vi "Process.vi"(8 "error in":errorcluster, 11 "Inst UI.MOTOR":refnum<class "Inst UI.MOTOR.lvclass">) -> (0 "error out":errorcluster, 3 "Inst UI.MOTOR out":refnum<class "Inst UI.MOTOR.lvclass">)   [LabVIEW 2019, in "Inst UI.MOTOR.lvclass"]
doc: "---------------------------------------------------------------\nJKI State Machine Objects™\nhttp://jki.net/state-machine-objects/\nCopyright (C) 2005-2015, JKI <info@jki.net>\nALL RIGHTS RESERVEDJKI State Machine Objects (SMO) 1.0.0.5\nJKI - JKI\nCopyright (c) 2016, JKI"
uses:
  Inst UI.MOTOR.lvclass
  C:/Program Files (x86)/National Instruments/LabVIEW 2019/vi.lib/JKI/JKI SMO/SMO/SMO.lvclass
  C:/Program Files (x86)/National Instruments/LabVIEW 2019/user.lib/LevyLab/Instrument Framework/SMOs/Instrument UI/Instrument UI.lvclass
  C:/Program Files (x86)/National Instruments/LabVIEW 2019/vi.lib/JKI/JKI SMO/SMO.UI/SMO.UI.lvclass
  Motor/Serial - XON-XOFF Characters.ctl
  Motor/Serial - ASCII Characters.ctl
  Inst.MOTOR/Typedefs/Inst.MOTOR.Commands--Enum.ctl
  Inst.MOTOR/Typedefs/Inst.MOTOR.getAll--Cluster.ctl
  Inst.MOTOR/Inst.MOTOR.lvclass
  C:/Program Files (x86)/National Instruments/LabVIEW 2019/user.lib/LevyLab/Instrument Framework/SMOs/Instrument/Instrument.lvclass
  Inst UI.MOTOR.UI--Cluster.ctl
  <userlib>/LevyLab/Instrument Framework/SMOs/Configuration/Configuration.lvclass
  <userlib>/LevyLab/Instrument Framework/SMOs/RemoteControl/Typedefs/Message--Cluster.ctl
  Inst.MOTOR/Typedefs/Inst.MOTOR.Configuration--Cluster.ctl
  <userlib>/LevyLab/Instrument Framework/SMOs/Instrument UI/Instrument UI.lvclass/Instrument UI.ctl
  Inst.MOTOR/Inst.MOTOR.lvclass/Inst.MOTOR.ctl
  <vilib>/JKI/JKI SMO/SMO/SMO.lvclass/SMO.ctl
  <userlib>/LevyLab/Instrument Framework/SMOs/Configuration/Configuration.lvclass/Configuration.ctl
  <userlib>/LevyLab/Instrument Framework/SMOs/Instrument/Instrument.lvclass/Instrument.ctl
  <userlib>/LevyLab/Instrument Framework/SMOs/Instrument/Typedefs/Client Type--Enum.ctl
  09e9697b-516c-49fb-b2dc-692589121b6f.vi
  <vilib>/JKI/JKI SMO/SMO/Private/ReftoDVR--SMO.vi
  09e9697b-516c-49fb-b2dc-692589121b6f.vi/bd16e97c-1283-4bf0-81fa-9ddf6985c1ae.vi
  09e9697b-516c-49fb-b2dc-692589121b6f.vi/bd16e97c-1283-4bf0-81fa-9ddf6985c1ae.vi/4ce74e04-6dcf-45ed-9e3a-8688fabe3fd2.vi
  <userlib>/LevyLab/Instrument Framework/SMOs/Instrument/API/Send and Receive.vi
  09e9697b-516c-49fb-b2dc-692589121b6f.vi/bd16e97c-1283-4bf0-81fa-9ddf6985c1ae.vi/122f345b-9992-4887-9e4c-64365b80683c.vi
  <userlib>/LevyLab/Instrument Framework/SMOs/Instrument/Private/Get Client Type.vi
  09e9697b-516c-49fb-b2dc-692589121b6f.vi/bd16e97c-1283-4bf0-81fa-9ddf6985c1ae.vi/4ce74e04-6dcf-45ed-9e3a-8688fabe3fd2.vi/d12c5baa-aee5-401d-8272-1247450cc591.vi
  09e9697b-516c-49fb-b2dc-692589121b6f.vi/bd16e97c-1283-4bf0-81fa-9ddf6985c1ae.vi/4ce74e04-6dcf-45ed-9e3a-8688fabe3fd2.vi/9d50bdb1-c95d-42e6-b665-6d4980af7bdd.vi
  09e9697b-516c-49fb-b2dc-692589121b6f.vi/bd16e97c-1283-4bf0-81fa-9ddf6985c1ae.vi/122f345b-9992-4887-9e4c-64365b80683c.vi/c58dab05-969e-483a-9f90-fe9d022133c9.vi
  09e9697b-516c-49fb-b2dc-692589121b6f.vi/bd16e97c-1283-4bf0-81fa-9ddf6985c1ae.vi/122f345b-9992-4887-9e4c-64365b80683c.vi/09663c29-364a-4026-bee6-568e439f1e9d.vi
  09e9697b-516c-49fb-b2dc-692589121b6f.vi/bd16e97c-1283-4bf0-81fa-9ddf6985c1ae.vi/122f345b-9992-4887-9e4c-64365b80683c.vi/c58dab05-969e-483a-9f90-fe9d022133c9.vi/7baa1985-5e51-47ea-8afb-6dd3369df49d.vi
  09e9697b-516c-49fb-b2dc-692589121b6f.vi/bd16e97c-1283-4bf0-81fa-9ddf6985c1ae.vi/122f345b-9992-4887-9e4c-64365b80683c.vi/c58dab05-969e-483a-9f90-fe9d022133c9.vi/1d83d098-8c96-44ae-b21b-eeb7af13dafe.vi
  <userlib>/LevyLab/Instrument Framework/SMOs/Instrument/Private/Get RC Connection Status.vi
  <userlib>/LevyLab/Instrument Framework/SMOs/RemoteControl/API/Send and Receive.vi
  <vilib>/Utility/Data Type/Get Type Information.vi
  <vilib>/JDP Science/JSONtext/JSON text to Variant.vi
  <vilib>/JDP Science/JSONtext/Variant to JSON Text.vi
  <vilib>/National Instruments/GUID Generator/Guid Generator.vi
  <userlib>/LevyLab/Instrument Framework/SMOs/Instrument/Private/Instrument.MessageFromProcess.EventStructure.vi
  <userlib>/LevyLab/Instrument Framework/SMOs/Instrument/Instrument.lvclass
  <vilib>/JDP Science/JSONtext/LVClass Serializer/JSONtext LVClass Serializer.lvclass
  <userlib>/LevyLab/Instrument Framework/SMOs/Instrument UI/Instrument UI.lvclass
  <vilib>/JKI/JKI SMO/SMO/SMO.lvclass
  <vilib>/JKI/JKI SMO/SMO.UI/SMO.UI.lvclass
  <userlib>/LevyLab/Instrument Framework/SMOs/RemoteControl/RemoteControl.lvclass
  C:/Program Files (x86)/National Instruments/LabVIEW 2019/user.lib/LevyLab/Instrument Framework/Instrument Types/VSource/Instrument.VSource.lvclass
panel:
  out "Encoder Position":string
  in  "Tab Control":T1(tab)
  in  "Encoder Position":bool
  in  "Choose wfm":string(combo)
  in  "Stop Motor":bool
  in  "Set Encoder Data":bool
  in  "Set Jog":bool
  in  "wfmStep":i32
  in  "uStep":i32
  in  "Speed":i32
  in  "Angle":i32
  in  "Target Mode":bool
  in  "Speed":i32
  in  "Write Command":string="*IDN?"
  in  "Write":bool
  in  "Read":bool
  out "coerced(x)":u32
  out "Response":string
  in  "XON/XOFF Characters":T2={"XON"=enum."DC1", "XOFF"=enum."DC3"}
  in  "STOP":bool
  # "MOTOR"
  # "For instructions on how to use the JKI State Machine Objects, examples and video tutorials, visit:\nhttp://jki.net/state-machine-objects/\n\nJKI State Machine Objects™\nhttp://jki.net/state-machine-objects/\nCopyright (C) 2005-2015, JKI <info@jki.net>\nALL RIGHTS RESERVED"
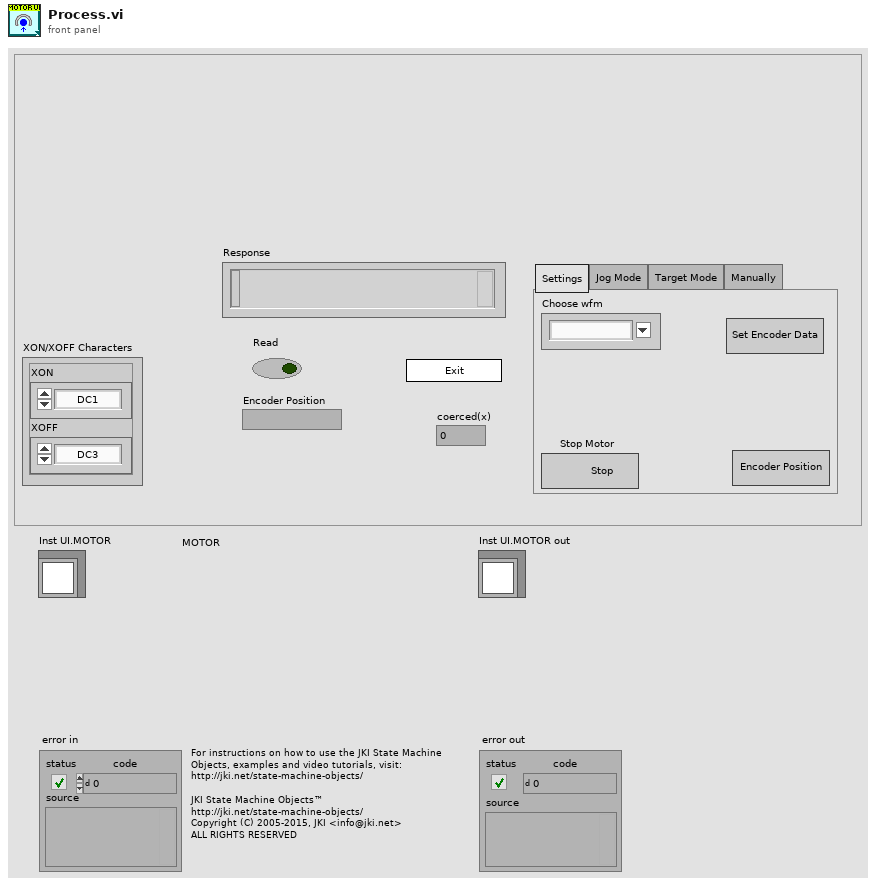
[diagram p1: front panel]
types:
  T1 = enum32{"Settings", "Jog Mode", "Target Mode", "Manually"}
  T2 = typedef "Serial - XON-XOFF Characters.ctl" = cluster{"XON":T3, "XOFF":T3}
  T3 = typedef "Serial - ASCII Characters.ctl" = enum16{"NUL", "SOH", "STX", "ETX", "EOT", "ENQ", "ACK", "BEL", "BS", "HT", "LF", "VT", "FF", "CR", "SO", "SI", "DLE", "DC1", "DC2", "DC3", "DC4", "NAK", "SYN", "ETB", "CAN", "EM", "SUB", "ESC", "FS", "GS", "RS", "US", "SP", "!", "\"", "#", "$", "%", "&", "'", "(", ")", "*", "+", ",", "- (-)", ".", "/", "0", "1", "2", "3", "4", "5", "6", "7", "8", "9", ":", ";", "<", "=", ">", "?", "@", "A", "B", "C", "D", "E", "F", "G", "H", "I", "J", "K", "L", "M", "N", "O", "P", "Q", "R", "S", "T", "U", "V", "W", "X", "Y", "Z", "[", "\\", "]", "^", "_", "`", "a", "b", "c", "d", "e", "f", "g", "h", "i", "j", "k", "l", "m", "n", "o", "p", "q", "r", "s", "t", "u", "v", "w", "x", "y", "z", "{", "|", "}", "~"}
  T4 = typedef "Inst.MOTOR.lvclass/Inst.MOTOR.Commands--Enum.ctl" = enum16{"Encoder Position", "VISA Read", "VISA Write"}
  T5 = enum32{"invalid app kind", "Development System", "Run Time System", "Student Edition", "Embedded LabVIEW", "Evaluation", "Custom"}
  T6 = enum32{"Invalid", "Standard", "Closed", "Hidden", "Minimized", "Maximized"}
  T7 = typedef "Instrument.lvclass/Client Type--Enum.ctl" = enum16{"Remote", "Local"}
  T8 = typedef "RemoteControl.lvclass/Message--Cluster.ctl" = cluster{"Command":string, "Data":variant, "ID":string}
  T9 = typedef "Inst.MOTOR.lvclass/Inst.MOTOR.Configuration--Cluster.ctl" = cluster{"baud rate":u32, "data bits":u16, "parity":enum16{"None", "Odd", "Even", "Mark", "Space"}, "stop bits":u16, "flow control":u16, "Read Count":u32, "Address":refnum<visa-resource-name>, "Termination Character":u8}
  T10 = typedef "Inst.MOTOR.lvclass/Inst.MOTOR.getAll--Cluster.ctl" = cluster{"Response":string, "Forward":bool, "Stop Motor":bool, "Encoder Position":string}
  T11 = typedef "Inst UI.MOTOR.lvclass/Inst UI.MOTOR.UI--Cluster.ctl" = cluster{" Read":string, "VISA resource name":refnum<visa-resource-name>}
  T12 = cluster{"Core":cluster{"Current VI Reference":refnum<vi>, "Close Panel on Exit?":bool, "Last Error":cluster{"error":errorcluster, "previous state":string, "remaining states":string}, "Shutdown?":bool}, "Instrument UI":refnum<class "Inst UI.MOTOR.lvclass">, "Instrument":refnum<class "Inst.MOTOR.lvclass">, "Configuration":refnum<class "Configuration.lvclass">, "Config Cluster":T9, "getAll":T10, "UI Cluster":T11, "Message":T8}
  T13 = cluster{"Current VI Reference":refnum<vi>, "Close Panel on Exit?":bool, "Last Error":cluster{"error":errorcluster, "previous state":string, "remaining states":string}, "Shutdown?":bool}
  T14 = typedef "SMO.lvclass/Protected Events.ctl" = cluster{"StopProcesses":refnum<user-event>, "AbortProcesses":refnum<user-event>, "Config Changed":refnum<user-event>, "Dependency":refnum<user-event>}
  T15 = typedef "Instrument.lvclass/PublicEvents--Cluster.ctl" = cluster{"MessageFromProcess":refnum<user-event>}
  T16 = typedef "Inst.MOTOR.lvclass/PublicEvents--Cluster.ctl" = cluster{"MessageFromProcess":refnum<user-event>}
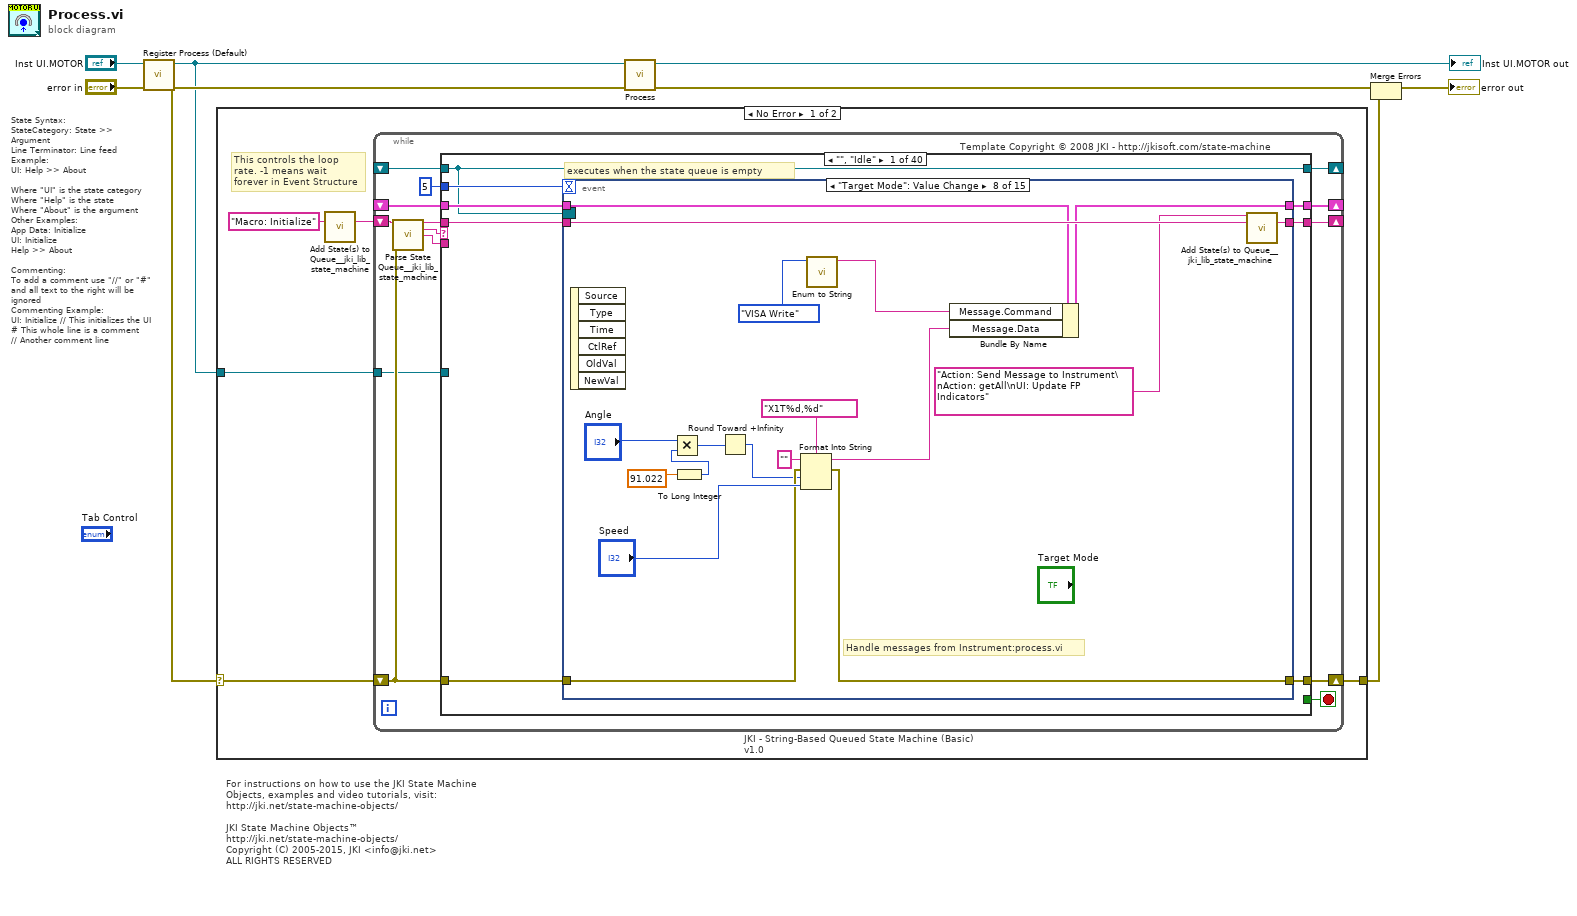
[diagram p0: block diagram]
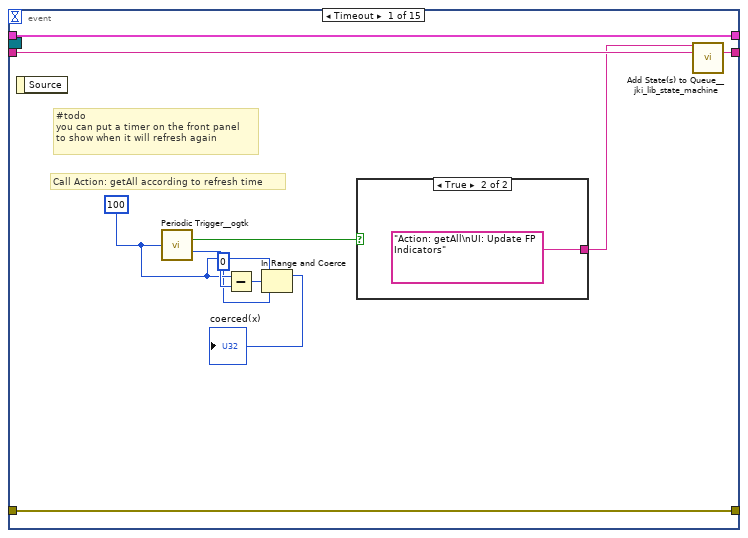
[diagram p2: hidden frame]
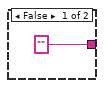
[diagram p3: hidden frame]
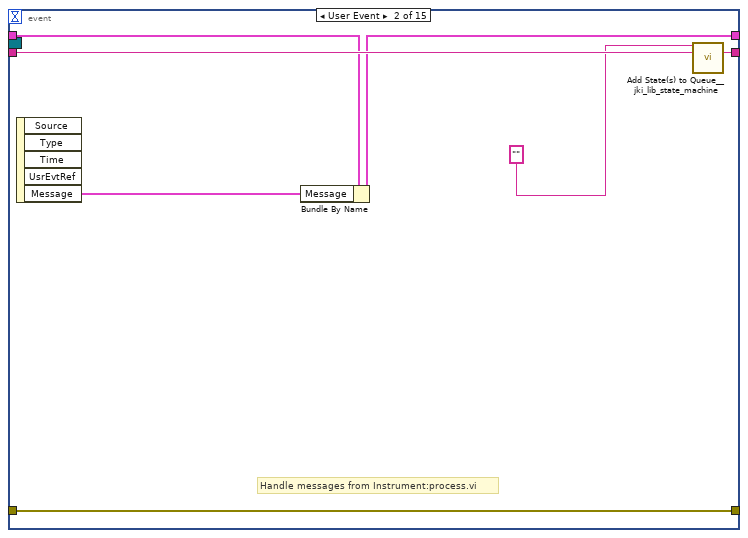
[diagram p4: hidden frame]
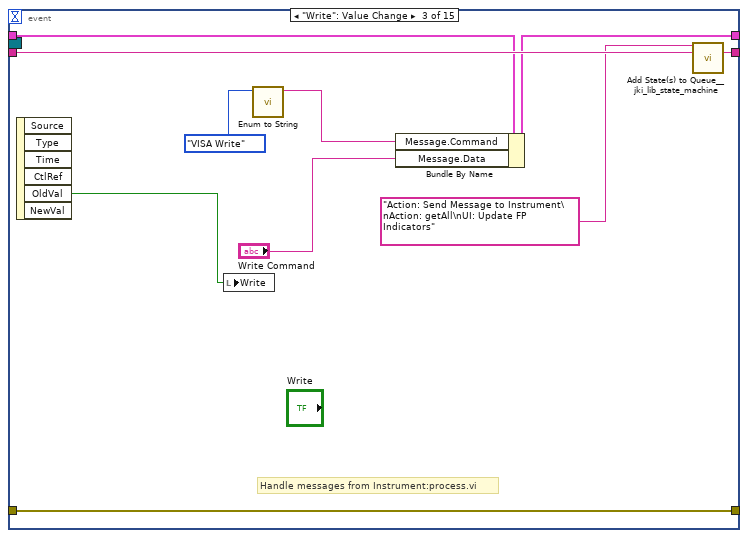
[diagram p5: hidden frame]
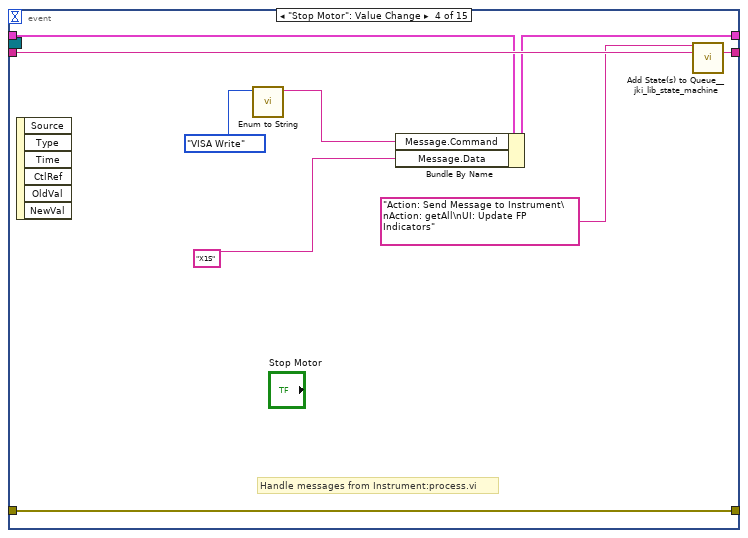
[diagram p6: hidden frame]
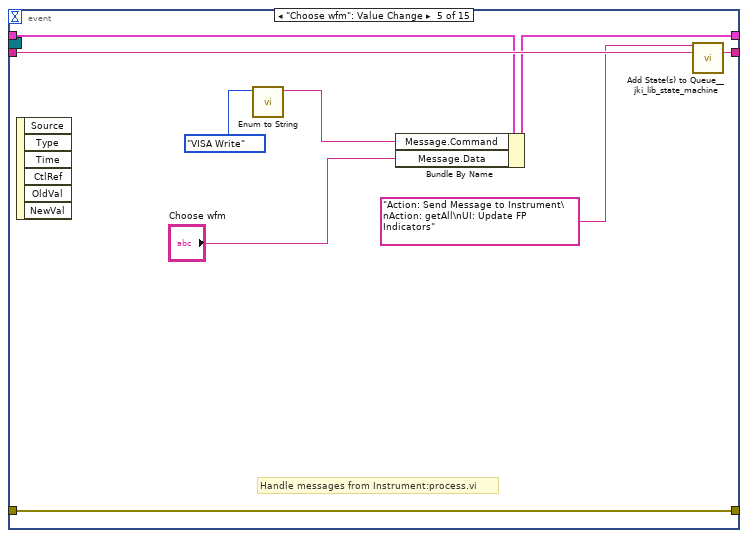
[diagram p7: hidden frame]
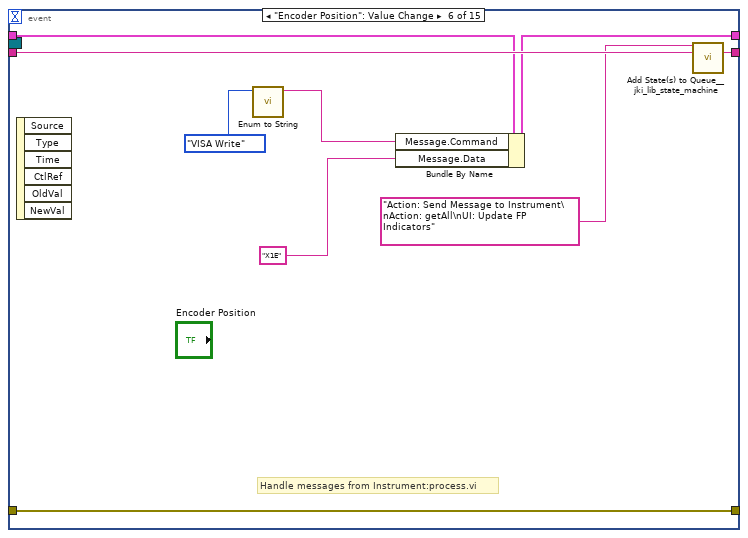
[diagram p8: hidden frame]
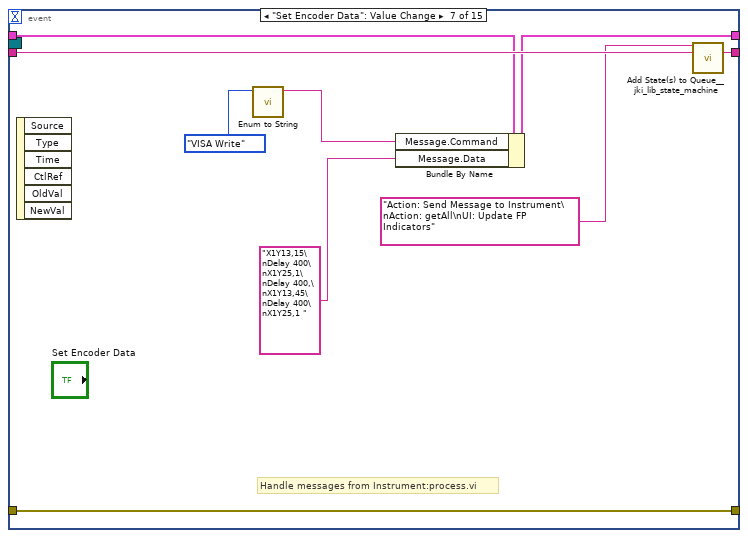
[diagram p9: hidden frame]
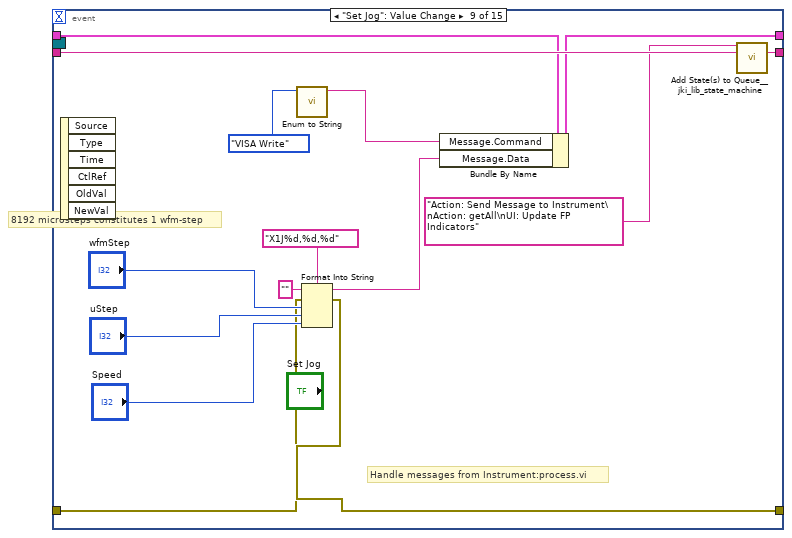
[diagram p10: hidden frame]
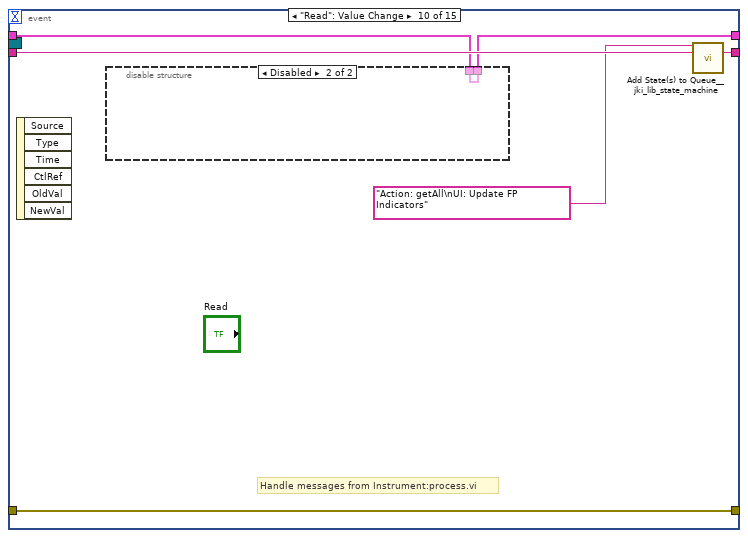
[diagram p11: hidden frame]
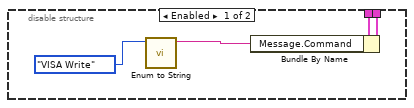
[diagram p12: hidden frame]
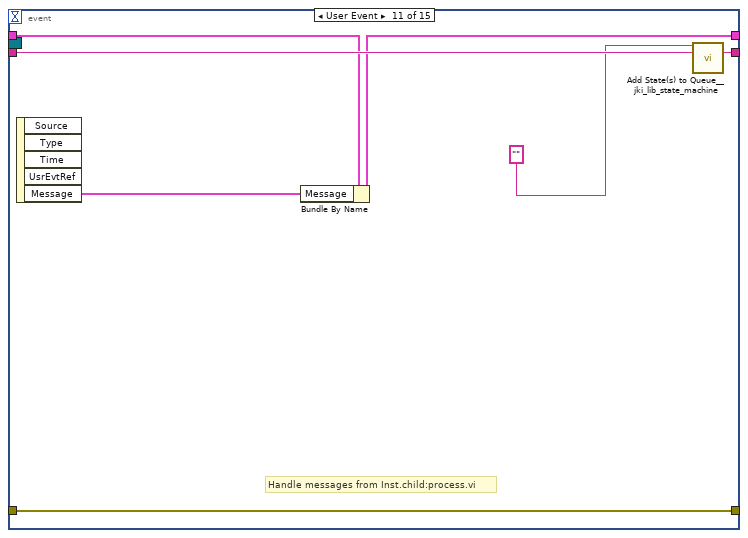
[diagram p13: hidden frame]
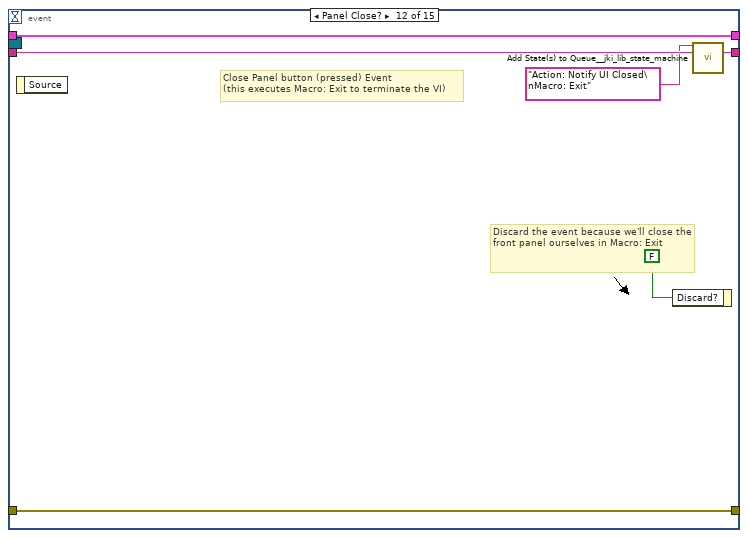
[diagram p14: hidden frame]
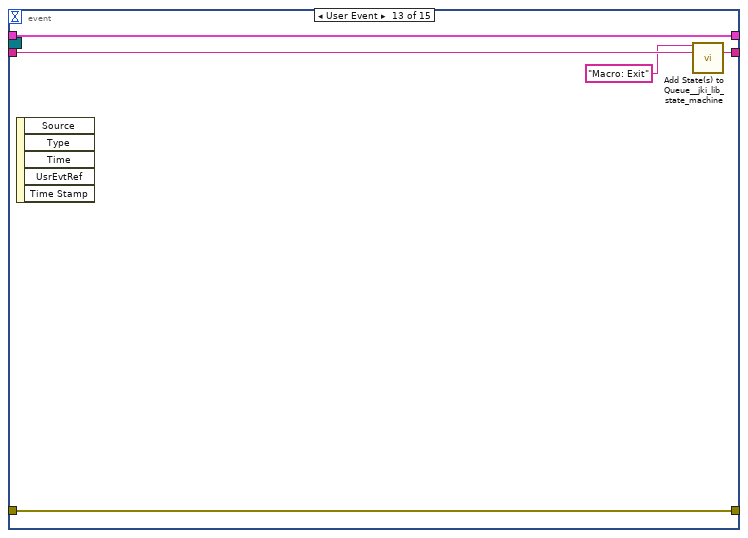
[diagram p15: hidden frame]
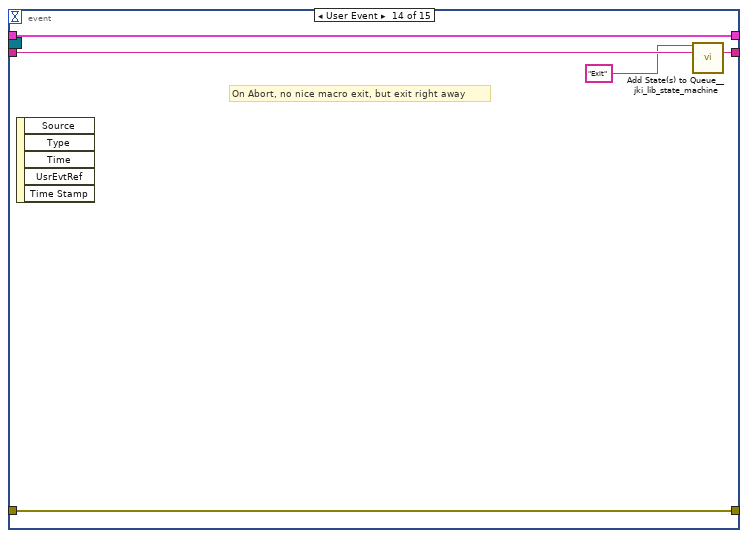
[diagram p16: hidden frame]
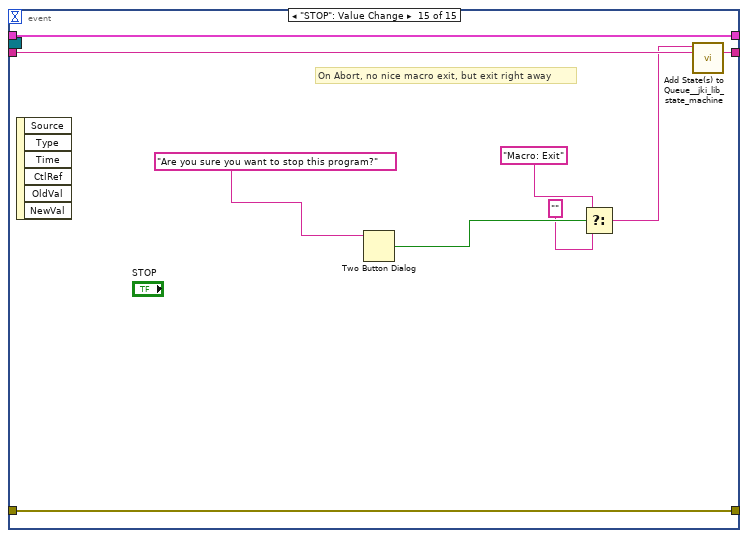
[diagram p17: hidden frame]
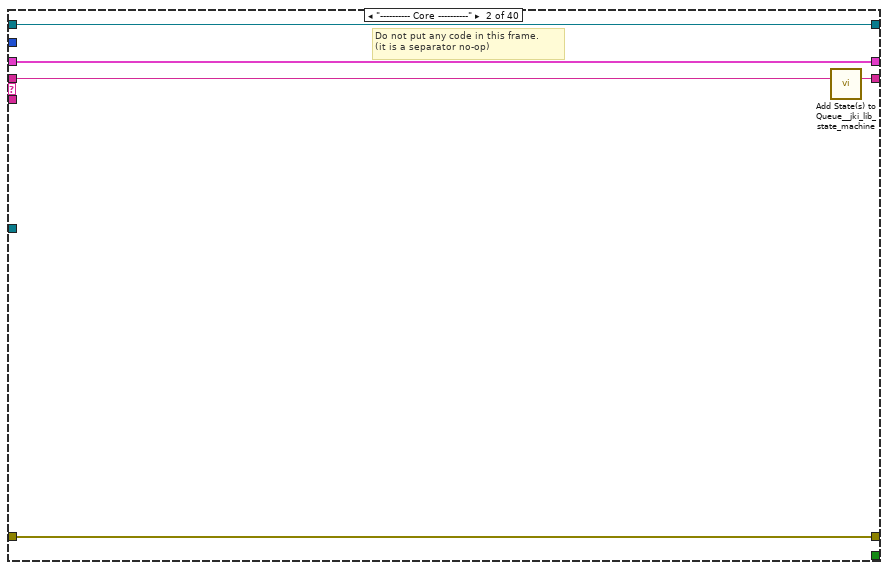
[diagram p18: hidden frame]
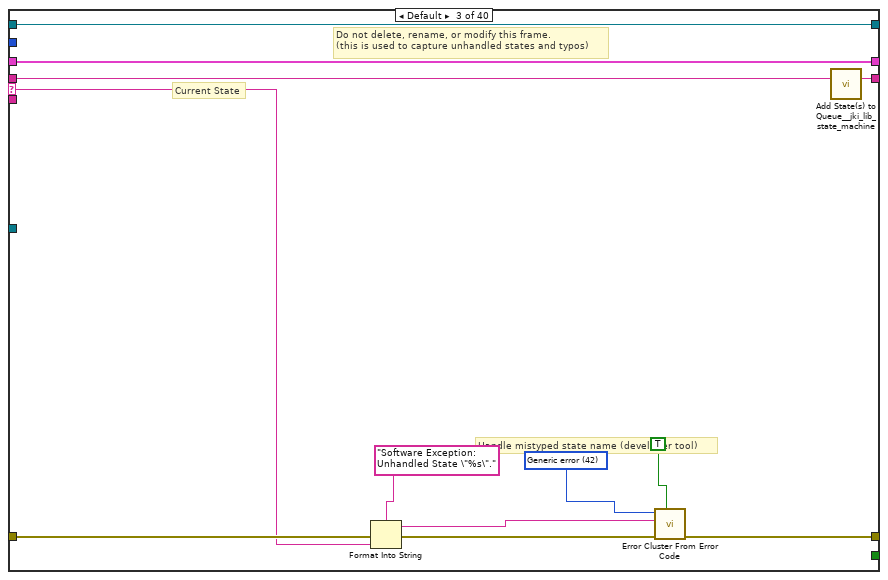
[diagram p19: hidden frame]
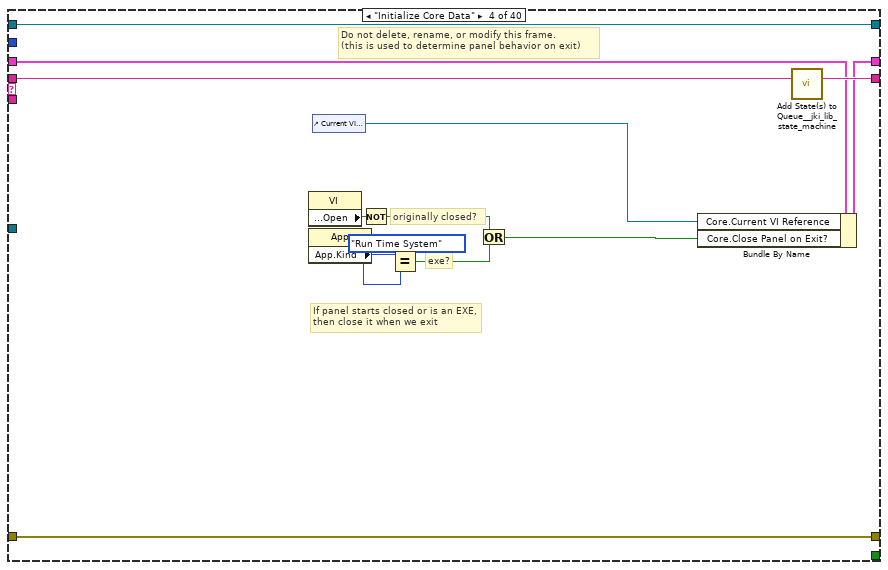
[diagram p20: hidden frame]
diagram:
  # "State Syntax:\nStateCategory: State >> Argument\nLine Terminator: Line feed\nExample:\nUI: Help >> About\n\nWhere \"UI\" is the state category\nWhere \"Help\" is the state\nWhere \"About\" is the argument\nOther Examples:\nApp Data: Initialize\nUI: Initialize\nHelp >> About\n\nCommenting:\nTo add a comment use \"//\" or \"#\" and all text to the right will be ignored\nCommenting Example:\nUI: Initialize // This initializes the UI\n# This whole line is a comment\n// Another comment line"
  # "For instructions on how to use the JKI State Machine Objects, examples and video tutorials, visit:\nhttp://jki.net/state-machine-objects/\n\nJKI State Machine Objects™\nhttp://jki.net/state-machine-objects/\nCopyright (C) 2005-2015, JKI <info@jki.net>\nALL RIGHTS RESERVED"
  n1 = call <vilib>:"Register Process (Default).vi"("error in (no error)"="error in", "SMO"="Inst UI.MOTOR") -> ("error out"=w5:errorcluster, "SelfRef"=w4:refnum<class "Inst UI.MOTOR.lvclass">)  [unwired: 8 in]
  n2 = case shown="No Error" w5 {
    selector: w5 -> [w10 w564]
    tunnel: w4 -> [w11 _]
    tunnel: [w9 w564] -> w1
    frame No Error {
      # "This controls the loop rate. -1 means wait forever in Event Structure"
      n3 = call <vilib>:"Add State(s) to Queue__jki_lib_state_machine.vi"("State(s) in (\"\")"="Macro: Initialize") -> ("States Out"=w13:string)  [unwired: 14 in]
      n4 = while "JKI - String-Based Queued State Machine (Basic) v1.0" {
        shift-right: [w20] -> _
        shift-left: _ -> [w19]
        shift-right: [w23] -> w9
        shift-left: w10 -> [w17]
        shift-right: [w22] -> _
        shift-left: w13 -> [w24]
        tunnel: w11 -> [w16]
        shift-right: [w15] -> _
        shift-left: _ -> [w14]
        stop <- w21 stop-if-true
        # "Template Copyright © 2008 JKI - http://jkisoft.com/state-machine"
        n5 = call <vilib>:"Parse State Queue__jki_lib_state_machine.vi"("State Queue"=w24, "Error In (no error)"=w17) -> ("Remaining States"=w26:string, "Current State"=w27:string, "Arguments"=w25:string)  [unwired: 11 in]
        n6 = case shown="\"\", \"Idle\"" w27 {
          selector: w27 -> [_ _ w184 _ _ _ _ _ _ _ _ _ _ _ _ _ _ _ _ _ _ _ _ _ _ _ _ _ _ _ _ _ _ _ _ _ _ _ _ _]
          tunnel: w26 -> [w35 w182 w188 w207 w211 w226 w231 w249 w254 w262 w269 w274 w281 w286 w295 w302 w318 w350 w359 w371 w381 w387 w402 w407 w418 w425 w430 w446 w452 w457 w472 w480 w492 w499 w506 w518 w531 w541 w553 w563]
          tunnel: w25 -> [_ _ _ _ _ _ _ _ _ _ _ _ _ _ _ w296 w312 _ _ _ _ _ _ _ _ _ _ _ _ _ _ _ _ _ _ _ _ _ _ _]
          tunnel: w19 -> [w33 w179 w186 w198 w214 w222 w228 _ w250 w258 w263 w271 w279 w283 w291 w300 w314 w347 w355 w361 w378 w384 w389 w404 w415 w420 w427 w444 w450 w454 w465 w477 w483 w494 w500 w510 w525 w533 w548 w558]
          tunnel: [w32 w180 w190 w204 w216 w221 w229 w238 w252 w260 w265 w272 w276 w282 w292 w297 w315 w348 w357 w369 w379 w385 w400 w405 w409 w421 w428 w441 w447 w455 w458 w475 w484 w496 w501 w515 w528 w538 w544 w554] -> w23
          tunnel: w17 -> [w31 w180 w189 w204 w210 _ w229 w235 w252 w260 w266 w272 w277 w282 w292 w298 w316 w348 w357 w369 w379 w385 w400 w405 w410 w422 w428 w431 w448 w455 w467 w473 w485 w496 w502 w511 w520 w534 w545 w555]
          tunnel: [w34 w181 w187 w206 w208 w225 w230 w248 w253 w261 w268 w273 w280 w285 w294 w301 w317 w349 w358 w370 w380 w386 w401 w406 w417 w424 w429 w445 w451 w456 w471 w479 w491 w498 w505 w517 w530 w540 w552 w562] -> w22
          tunnel: [_ _ _ _ _ TRUE _ _ _ _ _ _ _ _ _ _ _ _ _ _ _ _ _ _ _ _ _ _ _ _ _ _ _ _ _ _ _ _ _ _] -> w21
          tunnel: [w30 w179 w186 w205 w213 w222 w228 w247 w250 w258 w263 w271 w279 w283 w291 w300 w314 w347 w355 w362 w378 w384 w389 w404 w415 w420 w427 w444 w450 w454 w469 w477 w481 w493 w500 w512 w526 w535 w549 w559] -> w20
          tunnel: 5 ("Timeout") -> [w29 _ _ _ _ _ _ _ _ _ _ _ _ _ _ _ _ _ _ _ _ _ _ _ _ _ _ _ _ _ _ _ _ _ _ _ _ _ _ _]
          tunnel: w16 -> [_ _ _ _ _ _ _ w236 _ _ _ _ _ _ _ _ _ _ _ _ _ _ _ _ _ _ _ _ _ _ _ _ _ _ _ _ _ _ _ _]
          tunnel: [w28 w178 w183 w195 w220 w223 w227 w246 w251 w259 w264 w270 w278 w284 w293 w299 w311 w346 w356 w368 w377 w383 w394 w403 w416 w423 w426 w443 w449 w453 w470 w478 w490 w497 w504 w516 w529 w539 w551 w561] -> w15
          tunnel: w14 -> [w28 w178 w183 w195 w220 w223 w227 w246 w251 w259 w264 w270 w278 w284 w293 w299 w311 w346 w356 w368 w377 w383 w394 w403 w416 w423 w426 _ w449 w453 w470 w478 w490 w497 w504 w516 w529 w539 w551 w561]
          frame "", "Idle" {
            # "executes when the state queue is empty"
            n7 = event shown="[7] \"Target Mode\": Value Change" {
              selector: w28 -> [_ _ _ _ _ _ _ _ _ _ _ _ _ _ _]
              dyn-events: _ -> [_ _ _ _ _ _ _ _ _ _ _ _ _ _ _]
              timeout: w29 -> [_ _ _ _ _ _ _ _ _ _ _ _ _ _ _]
              tunnel: w35 -> [w46 w55 w65 w74 w83 w92 w101 w119 w134 w140 w152 w158 w163 w168 w177]
              tunnel: [w45 w54 w64 w73 w82 w91 w100 w118 w133 w139 w151 w157 w162 w167 w176] -> w34
              tunnel: w33 -> [w43 w52 w61 w70 w79 w88 w97 w116 w131 w135 w150 w154 w160 w165 w174]
              tunnel: [w44 w53 w63 w72 w81 w90 w99 w108 w122 w138 w146 w153 w161 w166 w175] -> w32
              tunnel: w31 -> [w44 w53 w63 w72 w81 w90 w99 w107 w121 w138 w146 w153 w161 w166 w175]
              tunnel: [w43 w51 w62 w71 w80 w89 w98 w117 w132 w136 w149 w154 w160 w165 w174] -> w30
              event Timeout {
                w38 = u32 100 ("time (ms)")
                # "#todo\nyou can put a timer on the front panel\nto show when it will refresh again"
                # "Call Action: getAll according to refresh time"
                n8 = event-data() -> ()  [unwired: 1 in, 1 out]
                n9 = call <userlib>:"Periodic Trigger__ogtk.vi"("time (ms)"=w38) -> ("Triggered"=w41:bool, "timer value"=w40:u32)  [unwired: 12 in, 1 out]
                n10 = Subtract(x=w38, y=w40) -> (x-y=w39:u32)
                n11 = In Range and Coerce(upper limit=w38, x=w39, lower limit=u32 0) -> (coerced(x)=→"coerced(x)":u32)  [unwired: 1 out]
                n12 = case shown="True" w41 {
                  tunnel: ["" ("State(s) in Front (\"\")") "Action: getAll\nUI: Update FP Indicators" ("State(s) in Front (\"\")")] -> w42
                  frame False {
                  }
                  frame True {
                  }
                }
                n13 = call <vilib>:"Add State(s) to Queue__jki_lib_state_machine.vi"("State(s) in Front (\"\")"=w42, "State(s) in (\"\")"=w46) -> ("States Out"=w45:string)  [unwired: 13 in]
              }
              event User Event {
                # "Handle messages from Instrument:process.vi"
                n14 = event-data() -> ("Message"=w49:T8)  [unwired: 1 in, 4 out]
                n15 = Bundle By Name(cluster=w52, "Message"=w49) -> (w51:T12)
                n16 = call <vilib>:"Add State(s) to Queue__jki_lib_state_machine.vi"("State(s) in Front (\"\")"="" ("State(s) in Front (\"\")"), "State(s) in (\"\")"=w55) -> ("States Out"=w54:string)  [unwired: 13 in]
              }
              event "Write": Value Change {
                # "Handle messages from Instrument:process.vi"
                n17 = event-data() -> ("OldVal"=w58:bool)  [unwired: 1 in, 5 out]
                n18 = local write "Write"(w58) -> ()
                n19 = call <userlib>:"Enum to String.vi"("Command"=Inst.MOTOR.Commands--Enum."VISA Write" ("Commands")) -> ("Command"=w59:string)  [unwired: 9 in, 1 out]
                n20 = Bundle By Name(cluster=w61, "Message.Command"=w59, "Message.Data"="Write Command") -> (w62:T12)
                n21 = call <vilib>:"Add State(s) to Queue__jki_lib_state_machine.vi"("State(s) in Front (\"\")"="Action: Send Message to Instrument\nAction: getAll\nUI: Update FP Indicators" ("State(s) in Front (\"\")"), "State(s) in (\"\")"=w65) -> ("States Out"=w64:string)  [unwired: 13 in]
              }
              event "Stop Motor": Value Change {
                # "Handle messages from Instrument:process.vi"
                n22 = event-data() -> ()  [unwired: 1 in, 6 out]
                n23 = call <userlib>:"Enum to String.vi"("Command"=Inst.MOTOR.Commands--Enum."VISA Write" ("Commands")) -> ("Command"=w69:string)  [unwired: 9 in, 1 out]
                n24 = Bundle By Name(cluster=w70, "Message.Command"=w69, "Message.Data"="X1S") -> (w71:T12)
                n25 = call <vilib>:"Add State(s) to Queue__jki_lib_state_machine.vi"("State(s) in Front (\"\")"="Action: Send Message to Instrument\nAction: getAll\nUI: Update FP Indicators" ("State(s) in Front (\"\")"), "State(s) in (\"\")"=w74) -> ("States Out"=w73:string)  [unwired: 13 in]
              }
              event "Choose wfm": Value Change {
                # "Handle messages from Instrument:process.vi"
                n26 = event-data() -> ()  [unwired: 1 in, 6 out]
                n27 = call <userlib>:"Enum to String.vi"("Command"=Inst.MOTOR.Commands--Enum."VISA Write" ("Commands")) -> ("Command"=w78:string)  [unwired: 9 in, 1 out]
                n28 = Bundle By Name(cluster=w79, "Message.Command"=w78, "Message.Data"="Choose wfm") -> (w80:T12)
                n29 = call <vilib>:"Add State(s) to Queue__jki_lib_state_machine.vi"("State(s) in Front (\"\")"="Action: Send Message to Instrument\nAction: getAll\nUI: Update FP Indicators" ("State(s) in Front (\"\")"), "State(s) in (\"\")"=w83) -> ("States Out"=w82:string)  [unwired: 13 in]
              }
              event "Encoder Position": Value Change {
                # "Handle messages from Instrument:process.vi"
                n30 = event-data() -> ()  [unwired: 1 in, 6 out]
                n31 = call <userlib>:"Enum to String.vi"("Command"=Inst.MOTOR.Commands--Enum."VISA Write" ("Commands")) -> ("Command"=w87:string)  [unwired: 9 in, 1 out]
                n32 = Bundle By Name(cluster=w88, "Message.Command"=w87, "Message.Data"="X1E") -> (w89:T12)
                n33 = call <vilib>:"Add State(s) to Queue__jki_lib_state_machine.vi"("State(s) in Front (\"\")"="Action: Send Message to Instrument\nAction: getAll\nUI: Update FP Indicators" ("State(s) in Front (\"\")"), "State(s) in (\"\")"=w92) -> ("States Out"=w91:string)  [unwired: 13 in]
              }
              event "Set Encoder Data": Value Change {
                # "Handle messages from Instrument:process.vi"
                n34 = event-data() -> ()  [unwired: 1 in, 6 out]
                n35 = call <userlib>:"Enum to String.vi"("Command"=Inst.MOTOR.Commands--Enum."VISA Write" ("Commands")) -> ("Command"=w96:string)  [unwired: 9 in, 1 out]
                n36 = Bundle By Name(cluster=w97, "Message.Command"=w96, "Message.Data"="X1Y13,15\nDelay 400\nX1Y25,1\nDelay 400,\nX1Y13,45\nDelay 400\nX1Y25,1 ") -> (w98:T12)
                n37 = call <vilib>:"Add State(s) to Queue__jki_lib_state_machine.vi"("State(s) in Front (\"\")"="Action: Send Message to Instrument\nAction: getAll\nUI: Update FP Indicators" ("State(s) in Front (\"\")"), "State(s) in (\"\")"=w101) -> ("States Out"=w100:string)  [unwired: 13 in]
              }
              event "Target Mode": Value Change {
                # "Handle messages from Instrument:process.vi"
                n38 = event-data() -> ()  [unwired: 1 in, 6 out]
                n39 = To Long Integer(number=91.022) -> (32bit integer=w103:i32)
                n40 = Multiply(x="Angle", y=w103) -> (x*y=w105:i32)
                n41 = Round Toward +Infinity(x=w105) -> (ceil(x): smallest int >= x=w104:i32)
                n42 = Format Into String(format string="X1T%d,%d", initial string="", error in=w107, w104, "Speed") -> (resulting string=w109:string, error out=w108:errorcluster)
                n43 = call <userlib>:"Enum to String.vi"("Command"=Inst.MOTOR.Commands--Enum."VISA Write" ("Commands")) -> ("Command"=w115:string)  [unwired: 9 in, 1 out]
                n44 = Bundle By Name(cluster=w116, "Message.Command"=w115, "Message.Data"=w109) -> (w117:T12)
                n45 = call <vilib>:"Add State(s) to Queue__jki_lib_state_machine.vi"("State(s) in Front (\"\")"="Action: Send Message to Instrument\nAction: getAll\nUI: Update FP Indicators" ("State(s) in Front (\"\")"), "State(s) in (\"\")"=w119) -> ("States Out"=w118:string)  [unwired: 13 in]
              }
              event "Set Jog": Value Change {
                # "8192 microsteps constitutes 1 wfm-step"
                # "Handle messages from Instrument:process.vi"
                n46 = event-data() -> ()  [unwired: 1 in, 6 out]
                n47 = call <userlib>:"Enum to String.vi"("Command"=Inst.MOTOR.Commands--Enum."VISA Write" ("Commands")) -> ("Command"=w130:string)  [unwired: 9 in, 1 out]
                n48 = Format Into String(format string="X1J%d,%d,%d", initial string="", error in=w121, "wfmStep", "uStep", "Speed") -> (resulting string=w120:string, error out=w122:errorcluster)
                n49 = Bundle By Name(cluster=w131, "Message.Command"=w130, "Message.Data"=w120) -> (w132:T12)
                n50 = call <vilib>:"Add State(s) to Queue__jki_lib_state_machine.vi"("State(s) in Front (\"\")"="Action: Send Message to Instrument\nAction: getAll\nUI: Update FP Indicators" ("State(s) in Front (\"\")"), "State(s) in (\"\")"=w134) -> ("States Out"=w133:string)  [unwired: 13 in]
              }
              event "Read": Value Change {
                # "Handle messages from Instrument:process.vi"
                n51 = event-data() -> ()  [unwired: 1 in, 6 out]
                n52 = disable-structure shown="Disabled" {
                  disable-tunnel: [w144 w145] -> w136
                  disable-tunnel: w135 -> [w143 w145]
                  frame Enabled {
                    n53 = call <userlib>:"Enum to String.vi"("Command"=Inst.MOTOR.Commands--Enum."VISA Write" ("Commands")) -> ("Command"=w142:string)  [unwired: 9 in, 1 out]
                    n54 = Bundle By Name(cluster=w143, "Message.Command"=w142) -> (w144:T12)
                  }
                  frame Disabled {
                  }
                }
                n55 = call <vilib>:"Add State(s) to Queue__jki_lib_state_machine.vi"("State(s) in Front (\"\")"="Action: getAll\nUI: Update FP Indicators" ("State(s) in Front (\"\")"), "State(s) in (\"\")"=w140) -> ("States Out"=w139:string)  [unwired: 13 in]
              }
              event User Event {
                # "Handle messages from Inst.child:process.vi"
                n56 = event-data() -> ("Message"=w147:T8)  [unwired: 1 in, 4 out]
                n57 = Bundle By Name(cluster=w150, "Message"=w147) -> (w149:T12)
                n58 = call <vilib>:"Add State(s) to Queue__jki_lib_state_machine.vi"("State(s) in Front (\"\")"="" ("State(s) in Front (\"\")"), "State(s) in (\"\")"=w152) -> ("States Out"=w151:string)  [unwired: 13 in]
              }
              event Panel Close? {
                # "Discard the event because we'll close the front panel ourselves in Macro: Exit"
                # "Close Panel button (pressed) Event\n(this executes Macro: Exit to terminate the VI)"
                n59 = event-data() -> ()  [unwired: 1 in, 1 out]
                n60 = event-data("Discard?"=FALSE) -> ()  [unwired: 1 in, 1 out]
                n61 = call <vilib>:"Add State(s) to Queue__jki_lib_state_machine.vi"("State(s) in Front (\"\")"="Action: Notify UI Closed\nMacro: Exit", "State(s) in (\"\")"=w158) -> ("States Out"=w157:string)  [unwired: 13 in]
              }
              event User Event {
                n62 = event-data() -> ()  [unwired: 1 in, 5 out]
                n63 = call <vilib>:"Add State(s) to Queue__jki_lib_state_machine.vi"("State(s) in Front (\"\")"="Macro: Exit", "State(s) in (\"\")"=w163) -> ("States Out"=w162:string)  [unwired: 13 in]
              }
              event User Event {
                # "On Abort, no nice macro exit, but exit right away"
                n64 = event-data() -> ()  [unwired: 1 in, 5 out]
                n65 = call <vilib>:"Add State(s) to Queue__jki_lib_state_machine.vi"("State(s) in Front (\"\")"="Exit", "State(s) in (\"\")"=w168) -> ("States Out"=w167:string)  [unwired: 13 in]
              }
              event "STOP": Value Change {
                # "On Abort, no nice macro exit, but exit right away"
                n66 = event-data() -> ()  [unwired: 1 in, 6 out]
                n67 = Two Button Dialog(message="Are you sure you want to stop this program?") -> (T button?=w173:bool)  [unwired: 2 in]
                n68 = Select(t="Macro: Exit", s=w173, f="") -> (s? t:f=w169:string)
                n69 = call <vilib>:"Add State(s) to Queue__jki_lib_state_machine.vi"("State(s) in Front (\"\")"=w169, "State(s) in (\"\")"=w177) -> ("States Out"=w176:string)  [unwired: 13 in]
              }
            }
          }
          frame "---------- Core ----------" {
            # "Do not put any code in this frame.\n(it is a separator no-op)"
            n70 = call <vilib>:"Add State(s) to Queue__jki_lib_state_machine.vi"("State(s) in (\"\")"=w182) -> ("States Out"=w181:string)  [unwired: 14 in]
          }
          frame Default {
            w193 = 42 items=["No error", "Argument error", "Memory is full", "Out of zone", "End of file", "File already open", "Generic file I/O error", "File not found", "File permission error", "Disk is full", "Duplicate path", "Too many files open", "System feature not enabled", "Resource file not found", "Cannot add resource", "Resource not found", "Image not found", "Image memory error", "Pen does not exist", "Config type invalid", "Config token not found", "Config parse error", "Config memory error", "Bad external code format", "Bad external code offset", "External code not present", "Null window", "Destroy window error", "Null menu", "Print aborted", "Bad print record", "Print driver error", "Windows error during printing", "Memory error during printing", "Print dialog error", "Generic print error", "Invalid device refnum", "Device not found", "Device parameter error", "Device unit error", "Cannot open device", "Device call aborted", "Generic error", "Cancelled by user", "Object ID too low", "Object ID too high", "Object not in heap", "Unknown heap", "Unknown object (invalid DefProc)", "Unknown object (DefProc not in table)", "Message out of range", "Invalid (null) method", "Unknown message", "Manager call not supported", "Bad address", "Network operation in progress", "Network operation timed out", "Connection is busy", "Network attribute not supported", "Network error", "Address in use", "System out of memory", "Connection aborted", "Connection refused", "Not connected", "Already connected", "Connection closed", "Initialization error (interapplication manager)", "Bad occurrence", "Wait on unbound occurrence handler", "Occurrence queue overflow", "Datalog type conflict", "Unused", "Unrecognized type (interapplication manager)", "Memory corrupt", "Failed to make temporary DLL", "Old CIN version", "Drag socket not found", "Failed to load drop-object", "Failed to register OLE object", "Failed to release OLE object", "Format specifier type mismatch", "Unknown format specifier", "Too few format specifiers", "Too many format specifiers", "Scan failed", "Newer CIN version", "Error converting to variant", "Runtime menu error", "Password tampered", "Variant attribute not found", "Incompatible variant data type", "Event data is not available", "Event Store is not present", "Occurrence is not found", "Event Queue is not created", "Event info is not available", "Refnum passed is NULL", "Error retrieving Class GUID", "Error retrieving CoClass GUID", "Error retrieving TypeLib GUID.", "Bad built application magic bytes.", "Specific driver is different from the specific driver associated with the Logical Name.", "There is no session opened to the class driver.", "Max Error", "MAX - Error with config objects", "MAX - Error loading configuration", "MAX - Group not supported"]
            # "Current State"
            # "Do not delete, rename, or modify this frame.\n(this is used to capture unhandled states and typos)"
            # "Handle mistyped state name (developer tool)"
            n71 = Format Into String(format string="Software Exception: Unhandled State \"%s\"." ("message"), error in=w189, w184) -> (resulting string=w192:string, error out=w191:errorcluster)  [unwired: 1 in]
            n72 = call <vilib>:"Error Cluster From Error Code.vi"("show call chain? (False)"=TRUE, "error in (no error)"=w191, "error message (\"\")"=w192, "error code (0)"=w193) -> ("error out"=w190:errorcluster)  [unwired: 5 in]
            n73 = call <vilib>:"Add State(s) to Queue__jki_lib_state_machine.vi"("State(s) in (\"\")"=w188) -> ("States Out"=w187:string)  [unwired: 14 in]
          }
          frame "Initialize Core Data" {
            # "Do not delete, rename, or modify this frame.\n(this is used to determine panel behavior on exit)"
            # "originally closed?"
            # "exe?"
            # "If panel starts closed or is an EXE, then close it when we exit"
            n74 = property class="VI"() -> ("Front Panel.Open"=w203:bool)  [unwired: 2 in, 2 out]
            n75 = property class="App"() -> ("App.Kind"=w202:T5)  [unwired: 2 in, 2 out]
            n76 = control-ref of="Current VI Reference"() -> (w196:refnum<vi>)
            n77 = Not(x=w203) -> (.not. x?=w200:bool)
            n78 = Equal?(x=w202, y=T5."Run Time System" ("Application:Kind")) -> (x = y?=w199:bool)
            n79 = Or(x=w200, y=w199) -> (x .or. y?=w197:bool)
            n80 = Bundle By Name(cluster=w198, "Core.Current VI Reference"=w196, "Core.Close Panel on Exit?"=w197) -> (w205:T12)
            n81 = call <vilib>:"Add State(s) to Queue__jki_lib_state_machine.vi"("State(s) in (\"\")"=w207) -> ("States Out"=w206:string)  [unwired: 14 in]
          }
          frame "Error Handler" {
            w216 = errorcluster {"status"=FALSE, "code"=0, "source"=""}  # No error
            # "Overwrite this method to handle errors and pass to parent if not handled. Parent will fire a public event if the error is not handled up the chain of classes."
            # "Handle any errors here.\nYou can also output any states to clean-up after errors occur"
            n82 = Unbundle By Name(w214) -> ("Instrument UI"=w219:refnum<class "Inst UI.MOTOR.lvclass">)
            n83 = call-dynamic "Handle Error.vi"("Stop on Unhandled Error (T)"=FALSE, "error in"=w210, "SMO"=w219) -> ("handling error"=w217:errorcluster, "Unhandled error"=w215:errorcluster)  [unwired: 6 in, 1 out]
            n84 = Bundle By Name(cluster=w214, "Core.Last Error.remaining states"=w211, "Core.Last Error.error"=w215) -> (w213:T12)
            n85 = Select(t="Exit", s=w217, f="Macro: Post Error Handling") -> (s? t:f=w208:string)
          }
          frame "Exit" {
            # "Do not put any code in this frame.\n(No errors that occur here will be handled.)"
            n86 = Unbundle By Name(w222) -> ("Core.Last Error.error"=w221:errorcluster)
            n87 = call <vilib>:"Add State(s) to Queue__jki_lib_state_machine.vi"("State(s) in (\"\")"=w226) -> ("States Out"=w225:string)  [unwired: 14 in]
          }
          frame "---------- Data ----------" {
            # "Do not put any code in this frame.\n(It is a separator no-op. You can make a copy of this frame to create a new Data frame)"
            n88 = call <vilib>:"Add State(s) to Queue__jki_lib_state_machine.vi"("State(s) in (\"\")"=w231) -> ("States Out"=w230:string)  [unwired: 14 in]
          }
          frame "Data: Initialize" {
            (unwired) T9 {"baud rate"=9600, "data bits"=8, "parity"=enum."None", "stop bits"=10, "flow control"=0, "Read Count"=1000, "Address"="", "Termination Character"=10}  # Config Cluster
            w232 = T9 {"baud rate"=9600, "data bits"=8, "parity"=enum."None", "stop bits"=10, "flow control"=0, "Read Count"=1000, "Address"="", "Termination Character"=10}  # Config Cluster
            w234 = T8 {"Command"="", "Data"=variant, "ID"=""}  # Message
            w237 = refnum<class "Configuration.lvclass"> refnum  # Configuration
            w240 = T11 {" Read"="", "VISA resource name"=""}  # UI Cluster
            w242 = refnum<class "Inst.MOTOR.lvclass"> refnum  # Instrument
            w244 = T10 {"Response"="", "Forward"=FALSE, "Stop Motor"=FALSE, "Encoder Position"=""}  # getAll
            w245 = T13 {"Current VI Reference"=refnum, "Close Panel on Exit?"=FALSE, "Last Error"={"error"={"status"=FALSE, "code"=0, "source"=""}, "previous state"="", "remaining states"=""}, "Shutdown?"=FALSE}  # Core
            # "typedef from Child Instrument"
            # "Cluster of UI\ninformation you\nwant to save/load"
            # "Child Instrument"
            # "typedef from Child Instrument"
            # "do not delete - used by framework"
            # "Data names and types of shift register data are defined by this bundle."
            # "Initialize the shift-register data, here.\n(data names are defined by what you wire into the bundle function)"
            n89 = call <userlib>:"Read Instrument.vi"("error in (no error)"=w235, "Instrument UI in"=w236) -> ("error out"=w239:errorcluster, "Instrument"=w241:refnum<class "Instrument.lvclass">, "Instrument UI"=w243:refnum<class "Inst UI.MOTOR.lvclass">)  [unwired: 7 in]
            n90 = To More Specific Class(target class=w242, reference=w241, error in=w239) -> (specific class reference=w233:refnum<class "Inst.MOTOR.lvclass">, error out=w238:errorcluster)
            n91 = Bundle("Core"=w245, "Instrument UI"=w243, "Instrument"=w233, "Configuration"=w237, "Config Cluster"=w232, "getAll"=w244, "UI Cluster"=w240, "Message"=w234) -> (w247:T12)  [unwired: 1 in]
            n92 = call <vilib>:"Add State(s) to Queue__jki_lib_state_machine.vi"("State(s) in (\"\")"=w249) -> ("States Out"=w248:string)  [unwired: 14 in]
          }
          frame "Data: Set UI Cluster" {
            # "Do not put any code in this frame.\n(It is a separator no-op. You can make a copy of this frame to create a new Data frame)"
            n93 = disable-structure shown="Disabled" {
              frame Disabled {
                n94 = Unbundle By Name("XON/XOFF Characters") -> ("XON"=w256:T3, "XOFF"=w255:T3)
                n95 = Bundle By Name("XON"=w256, "XOFF"=w255) -> ()  [unwired: 1 in, 1 out]
              }
              frame Enabled {
              }
            }
            n96 = call <vilib>:"Add State(s) to Queue__jki_lib_state_machine.vi"("State(s) in (\"\")"=w254) -> ("States Out"=w253:string)  [unwired: 14 in]
          }
          frame "Data: Set Config Cluster" {
            # "Do not put any code in this frame.\n(It is a separator no-op. You can make a copy of this frame to create a new Data frame)"
            n97 = call <vilib>:"Add State(s) to Queue__jki_lib_state_machine.vi"("State(s) in (\"\")"=w262) -> ("States Out"=w261:string)  [unwired: 14 in]
          }
          frame "Data: Cleanup" {
            # "Cleanup any data and references, here.\n(this is called automatically, by the Macro: Exit)"
            n98 = Unbundle By Name(w263) -> ("Core.Current VI Reference"=w267:refnum<vi>)
            n99 = Close Reference(reference=w267, error in (no error)=w266) -> (error out=w265:errorcluster)
            n100 = call <vilib>:"Add State(s) to Queue__jki_lib_state_machine.vi"("State(s) in (\"\")"=w269) -> ("States Out"=w268:string)  [unwired: 14 in]
          }
          frame "---------- UI ----------" {
            # "Do not put any code in this frame.\n(It is a separator no-op. You can make a copy of this frame to create a new UI frame)"
            n101 = call <vilib>:"Add State(s) to Queue__jki_lib_state_machine.vi"("State(s) in (\"\")"=w274) -> ("States Out"=w273:string)  [unwired: 14 in]
          }
          frame "UI: Initialize" {
            # "size window to decoration box on front panel"
            # "Initialize the User Interface, here.\n(this is called automatically, by the Macro: Init)"
            n102 = invoke on="STOP" class="Bool (strict)" method="Reinit To Default"() -> ()  [unwired: 3 in, 3 out]
            n103 = call <userlib>:"Fit VI window to Largest Dec__ogtk.vi"("error in (no error)"=w277, "border spacing (2 px)"=0) -> ("error out"=w276:errorcluster)  [unwired: 4 in, 1 out]
            n104 = call <vilib>:"Add State(s) to Queue__jki_lib_state_machine.vi"("State(s) in (\"\")"=w281) -> ("States Out"=w280:string)  [unwired: 14 in]
          }
          frame "UI: Update FP Controls" {
            # "Do not put any code in this frame.\n(It is a separator no-op. You can make a copy of this frame to create a new UI frame)"
            n105 = call <vilib>:"Add State(s) to Queue__jki_lib_state_machine.vi"("State(s) in (\"\")"=w286) -> ("States Out"=w285:string)  [unwired: 14 in]
          }
          frame "UI: Update FP Indicators" {
            # "do this way to have nicer UI or only display what you want"
            n106 = Unbundle By Name(w291) -> ("getAll.Response"=→"Response":string, "getAll.Encoder Position"=w288:string)
            n107 = String Subset(string=w288, offset (0)=3) -> (substring=→"Encoder Position":string)  [unwired: 1 in]
            n108 = call <vilib>:"Add State(s) to Queue__jki_lib_state_machine.vi"("State(s) in (\"\")"=w295) -> ("States Out"=w294:string)  [unwired: 14 in]
          }
          frame "UI: Cursor Set" {
            # "Argument"
            # "Initialize the User Interface, here.\n(this is called automatically, by the Macro: Init)"
            n109 = disable-structure shown="Default" {
              disable-tunnel: w298 -> [w303 w306]
              disable-tunnel: [w303 w305] -> w297
              disable-tunnel: w296 -> [_ w304]
              frame condition #0 {
              }
              frame condition #1 (active) {
                n110 = case shown="\"Busy\"" w304 {
                  tunnel: w306 -> [w308 w310]
                  tunnel: [w307 w309] -> w305
                  frame "Idle", Default {
                    n111 = call <vilib>:"Unset Busy.vi"("error in (no error)"=w308) -> ("error out"=w307:errorcluster)  [unwired: 10 in]
                  }
                  frame "Busy" {
                    n112 = call <vilib>:"Set Busy.vi"("error in (no error)"=w310) -> ("error out"=w309:errorcluster)  [unwired: 9 in, 1 out]
                  }
                }
              }
            }
            n113 = call <vilib>:"Add State(s) to Queue__jki_lib_state_machine.vi"("State(s) in (\"\")"=w302) -> ("States Out"=w301:string)  [unwired: 14 in]
          }
          frame "UI: Front Panel State" {
            # "Argument"
            # "Set Front Panel Open or Closed\n(Usage: \"UI: Front Panel State >> Open|Close\")"
            n114 = Unbundle By Name(w314) -> ("Core.Current VI Reference"=w313:refnum<vi>)
            n115 = disable-structure shown="Default" {
              disable-tunnel: w316 -> [w322 w345]
              disable-tunnel: [w321 w345] -> w315
              disable-tunnel: w313 -> [w320 _]
              disable-tunnel: w312 -> [w319 _]
              frame condition #0 (active) {
                n116 = case shown="\"Close\"" w319 {
                  tunnel: w322 -> [w326 w339]
                  tunnel: [w328 w340] -> w321
                  tunnel: w320 -> [w327 w337]
                  frame "Open", Default {
                    n117 = property class="VI"(reference=w327, error in=w326) -> (reference out=w324:refnum<vi>, error out=w325:errorcluster, "FP.State"=w323:T6)
                    n118 = case shown="\"Closed\"" w323 {
                      tunnel: [w331 w334] -> w328
                      tunnel: w325 -> [w330 w334]
                      tunnel: w324 -> [w329 _]
                      frame "Closed" {
                        n119 = invoke class="VI" method="FP.Open"(reference=w329, error in=w330, "Activate"=TRUE, "State"=T6."Standard") -> (error out=w331:errorcluster)  [unwired: 1 in, 4 out]
                      }
                      frame Default {
                      }
                    }
                  }
                  frame "Close" {
                    n120 = property class="VI"(reference=w337, error in=w339) -> (reference out=w336:refnum<vi>, error out=w338:errorcluster, "FP.State"=w335:T6)
                    n121 = case shown="Default" w335 {
                      tunnel: [w341 w344] -> w340
                      tunnel: w338 -> [w341 w343]
                      tunnel: w336 -> [_ w342]
                      frame "Invalid", "Closed" {
                      }
                      frame Default {
                        n122 = invoke class="VI" method="FP.Close"(reference=w342, error in=w343) -> (error out=w344:errorcluster)  [unwired: 1 in, 2 out]
                      }
                    }
                  }
                }
              }
              frame condition #1 {
              }
            }
            n123 = call <vilib>:"Add State(s) to Queue__jki_lib_state_machine.vi"("State(s) in (\"\")"=w318) -> ("States Out"=w317:string)  [unwired: 14 in]
          }
          frame "---------- Macro ----------" {
            # "Do not put any code in this frame.\n(It is a separator no-op. You can make a copy of this frame to create a new Macro frame)"
            n124 = call <vilib>:"Add State(s) to Queue__jki_lib_state_machine.vi"("State(s) in (\"\")"=w350) -> ("States Out"=w349:string)  [unwired: 14 in]
          }
          frame "Macro: Initialize" {
            w353 = "UI: Initialize\nMacro: Read UI Config\nAction: Open\n//UI: Front Panel State >> Open"  # UI: Initialize Macro: Read UI Config Action: Open //UI: Front Panel State >> Open
            # "Initialization Macro\n(This is called once, when the VI starts)"
            n125 = call <vilib>:"Add State(s) to Queue__jki_lib_state_machine.vi"("State(s) in Front (\"\")"="Data: Initialize\nInitialize Core Data\nEvents: Register", "State(s) in (\"\")"="Process: Sync", "State(s) at Back (\"\")"=w353) -> ("States Out"=w352:string)  [unwired: 12 in]
            n126 = call <vilib>:"Add State(s) to Queue__jki_lib_state_machine.vi"("State(s) in Front (\"\")"=w352, "State(s) in (\"\")"=w359) -> ("States Out"=w358:string)  [unwired: 13 in]
          }
          frame "Macro: Post Error Handling" {
            # "Clear Last Error?"
            n127 = Unbundle By Name(w361) -> ("Core.Last Error.remaining states"=w363:string, "Core.Shutdown?"=w364:bool)
            n128 = Unbundle By Name(w361) -> ("Core.Last Error.error"=w367:errorcluster)
            n129 = case shown="False" FALSE {
              tunnel: w367 -> [w375 _]
              tunnel: [w375 _] -> w366
              frame False {
              }
              frame True {
              }
            }
            n130 = case shown="False" w364 {
              tunnel: w363 -> [w372 w374]
              tunnel: [w372 w373] -> w360
              frame False {
                # "These are the remaining states (at the moment the error occured). States can be altered according to business logic."
                # "NOT SHUTTING DOWN"
              }
              frame True {
                # "Developer can decide to alter the states but should be aware that during the shutdown process, there are certain states that must be run for the SMO to properly shut itself (and this process) down. As such, one can add states to perform additional clean-ups, but should append the remaining state to be executed."
                # "SHUTTING DOWN"
                n131 = call <vilib>:"Add State(s) to Queue__jki_lib_state_machine.vi"("State(s) in (\"\")"=w374) -> ("States Out"=w373:string)  [unwired: 14 in]
              }
            }
            n132 = Bundle By Name(cluster=w361, "Core.Last Error.error"=w366) -> (w362:T12)
            n133 = call <vilib>:"Add State(s) to Queue__jki_lib_state_machine.vi"("State(s) in Front (\"\")"=w360, "State(s) in (\"\")"=w371) -> ("States Out"=w370:string)  [unwired: 13 in]
          }
          frame "Macro: Read UI Config" {
            # "Do not put any code in this frame.\n(It is a separator no-op. You can make a copy of this frame to create a new Macro frame)"
            n134 = call <vilib>:"Add State(s) to Queue__jki_lib_state_machine.vi"("State(s) in Front (\"\")"="Configuration: Initialize\nConfiguration: Read UI Config File\nUI: Update FP Controls" ("State(s) in Front (\"\")"), "State(s) in (\"\")"=w381) -> ("States Out"=w380:string)  [unwired: 13 in]
          }
          frame "Macro: Write UI Config" {
            # "Do not put any code in this frame.\n(It is a separator no-op. You can make a copy of this frame to create a new Macro frame)"
            n135 = call <vilib>:"Add State(s) to Queue__jki_lib_state_machine.vi"("State(s) in Front (\"\")"="Data: Set UI Cluster\nConfiguration: Write UI Config File" ("State(s) in Front (\"\")"), "State(s) in (\"\")"=w387) -> ("States Out"=w386:string)  [unwired: 13 in]
          }
          frame "Macro: Exit" {
            # "Exit Macro\n(This is called once, when the VI exits)"
            n136 = Unbundle By Name(w389) -> ("Core.Close Panel on Exit?"=w399:bool)
            n137 = Select(t="UI: Front Panel State >> Close", s=w399, f="" ("Empty String Constant")) -> (s? t:f=w396:string)
            n138 = call <vilib>:"Add State(s) to Queue__jki_lib_state_machine.vi"("State(s) in Front (\"\")"="Data: Cleanup\nEvents: Unregister\nProcess: Self Terminate", "State(s) in (\"\")"="Process: Sync", "State(s) at Back (\"\")"="Exit") -> ("States Out"=w391:string)  [unwired: 12 in]
            n139 = call <vilib>:"Add State(s) to Queue__jki_lib_state_machine.vi"("State(s) in Front (\"\")"="Action: Close\nMacro: Write UI Config", "State(s) in (\"\")"=w396, "State(s) at Back (\"\")"=w391) -> ("States Out"=w395:string)  [unwired: 12 in]
            n140 = call <vilib>:"Add State(s) to Queue__jki_lib_state_machine.vi"("State(s) in Front (\"\")"=w395, "State(s) in (\"\")"=w402) -> ("States Out"=w401:string)  [unwired: 13 in]
          }
          frame "---------- Process ----------" {
            # "Template Separator\n(You can make a copy of, or modify, this frame)"
            n141 = call <vilib>:"Add State(s) to Queue__jki_lib_state_machine.vi"("State(s) in (\"\")"=w407) -> ("States Out"=w406:string)  [unwired: 14 in]
          }
          frame "Process: Sync" {
            n142 = Unbundle By Name(w415) -> ("Instrument UI"=w411:refnum<class "Inst UI.MOTOR.lvclass">)
            n143 = call <vilib>:"WaitOnProcessSync.vi"("error in (no error)"=w410, "SMO"=w411) -> ("error out"=w409:errorcluster, "Don't run?"=w414:bool)  [unwired: 7 in, 1 out]
            n144 = Select(t="Data: Cleanup\nEvents: Unregister\nExit", s=w414, f="" ("Empty String Constant")) -> (s? t:f=w408:string)
            n145 = call <vilib>:"Add State(s) to Queue__jki_lib_state_machine.vi"("State(s) in Front (\"\")"=w408, "State(s) in (\"\")"=w418) -> ("States Out"=w417:string)  [unwired: 13 in]
          }
          frame "Process: Self Terminate" {
            n146 = Unbundle By Name(w420) -> ("Instrument UI"=w419:refnum<class "Inst UI.MOTOR.lvclass">)
            n147 = call <vilib>:"SelfTerminate.vi"("error in (no error)"=w422, "SMO in"=w419) -> ("error out"=w421:errorcluster)  [unwired: 8 in, 1 out]
            n148 = call <vilib>:"Add State(s) to Queue__jki_lib_state_machine.vi"("State(s) in (\"\")"=w425) -> ("States Out"=w424:string)  [unwired: 14 in]
          }
          frame "---------- Events ----------" {
            # "Template Separator\n(You can make a copy of, or modify, this frame)"
            n149 = call <vilib>:"Add State(s) to Queue__jki_lib_state_machine.vi"("State(s) in (\"\")"=w430) -> ("States Out"=w429:string)  [unwired: 14 in]
          }
          frame "Events: Register" {
            # "Expand to add\nmore events"
            # "Base Class Protected Events"
            n150 = Unbundle By Name(w444) -> ("Instrument UI"=w437:refnum<class "Inst UI.MOTOR.lvclass">, "Instrument"=w436:refnum<class "Inst.MOTOR.lvclass">)
            n151 = call <vilib>:"GetProtectedEvents.vi"("SMO"=w437) -> ("error out"=w440:errorcluster, "SMO Protected Events"=w442:T14)  [unwired: 8 in, 1 out]
            n152 = call <userlib>:"Instrument.GetPublicEvents.vi"("Instrument"=w436) -> ("error out"=w438:errorcluster, "Instrument Public Events"=w439:T15, "Instrument out"=w434:refnum<class "Inst.MOTOR.lvclass">)  [unwired: 8 in]
            n153 = call "Inst.MOTOR.GetPublicEvents.vi"("Inst.MOTOR in"=w434) -> ("error out"=w433:errorcluster, "Inst.MOTOR Public Events"=w435:T16)  [unwired: 8 in, 1 out]
            n154 = register-events(w442, w439, w435) -> (reference out=w443:refnum<event-registration>, error out=w432:errorcluster)  [unwired: 2 in]
            n155 = Merge Errors(w432, w433, w438, w440, w431) -> (w441:errorcluster)
            n156 = call <vilib>:"Add State(s) to Queue__jki_lib_state_machine.vi"("State(s) in (\"\")"=w446) -> ("States Out"=w445:string)  [unwired: 14 in]
          }
          frame "Events: Unregister" {
            n157 = Unregister For Events(event registration refnum=w449, error in=w448) -> (error out=w447:errorcluster)
            n158 = call <vilib>:"Add State(s) to Queue__jki_lib_state_machine.vi"("State(s) in (\"\")"=w452) -> ("States Out"=w451:string)  [unwired: 14 in]
          }
          frame "---------- Configuration ----------" {
            # "Do not put any code in this frame.\n(It is a separator no-op. You can make a copy of this frame to create a new UI frame)"
            n159 = call <vilib>:"Add State(s) to Queue__jki_lib_state_machine.vi"("State(s) in (\"\")"=w457) -> ("States Out"=w456:string)  [unwired: 14 in]
          }
          frame "Configuration: Initialize" {
            # "Do not put any code in this frame.\n(It is a separator no-op. You can make a copy of this frame to create a new UI frame)"
            n160 = Unbundle By Name(w465) -> ("Configuration"=w463:refnum<class "Configuration.lvclass">, "Instrument"=w464:refnum<class "Inst.MOTOR.lvclass">)
            n161 = call <vilib>:"GetName.vi"("error in (no error)"=w467, "SMO"=w464) -> ("error out"=w466:errorcluster, "Name"=w468:string)  [unwired: 6 in, 2 out]
            n162 = call <userlib>:"Default Path.vi"("error in (no error)"=w466, "Folder Name [Application Name]"=w468, "Configuration in"=w463) -> ("error out"=w459:errorcluster, "Configuration out"=w462:refnum<class "Configuration.lvclass">)  [unwired: 7 in]
            n163 = call <userlib>:"Write Section.vi"("error in (no error)"=w459, "Section"="UI", "Configuration in"=w462) -> ("error out"=w458:errorcluster, "Configuration out"=w461:refnum<class "Configuration.lvclass">)  [unwired: 7 in]
            n164 = Bundle By Name(cluster=w465, "Configuration"=w461) -> (w469:T12)
            n165 = call <vilib>:"Add State(s) to Queue__jki_lib_state_machine.vi"("State(s) in (\"\")"=w472) -> ("States Out"=w471:string)  [unwired: 14 in]
          }
          frame "Configuration: Write UI Config File" {
            # "Do not put any code in this frame.\n(It is a separator no-op. You can make a copy of this frame to create a new Data frame)"
            n166 = Unbundle By Name(w477) -> ("Configuration"=w474:refnum<class "Configuration.lvclass">, "UI Cluster"=w476:T11)
            n167 = call <userlib>:"Write Configuration.vi"("error in (no error)"=w473, "Variant"=w476, "Configuration in"=w474) -> ("error out"=w475:errorcluster)  [unwired: 7 in, 1 out]
            n168 = call <vilib>:"Add State(s) to Queue__jki_lib_state_machine.vi"("State(s) in (\"\")"=w480) -> ("States Out"=w479:string)  [unwired: 14 in]
          }
          frame "Configuration: Read UI Config File" {
            # "Do not put any code in this frame.\n(It is a separator no-op. You can make a copy of this frame to create a new UI frame)"
            n169 = Unbundle By Name(w483) -> ("UI Cluster"=w486:T11, "Configuration"=w489:refnum<class "Configuration.lvclass">)
            n170 = call <userlib>:"Read Configuration.vi"("INI Fomatted Cluster Type"=w486, "error in (no error)"=w485, "Configuration in"=w489) -> ("error out"=w488:errorcluster, "Configuration"=w487:variant)  [unwired: 6 in, 1 out]
            n171 = Variant To Data(error in=w488, type=w486, Variant=w487) -> (data=w482:T11, error out=w484:errorcluster)
            n172 = Bundle By Name(cluster=w483, "UI Cluster"=w482) -> (w481:T12)
            n173 = call <vilib>:"Add State(s) to Queue__jki_lib_state_machine.vi"("State(s) in (\"\")"=w492) -> ("States Out"=w491:string)  [unwired: 14 in]
          }
          frame "---------- Action ----------" {
            n174 = Unbundle By Name(w494) -> ("Instrument"=w495:refnum<class "Inst.MOTOR.lvclass">)
            n175 = Bundle By Name(cluster=w494, "Instrument"=w495) -> (w493:T12)
            n176 = call <vilib>:"Add State(s) to Queue__jki_lib_state_machine.vi"("State(s) in (\"\")"=w499) -> ("States Out"=w498:string)  [unwired: 14 in]
          }
          frame "Action: Notify UI Closed" {
            # "Notify that the UI has been closed"
            n177 = Unbundle By Name(w500) -> ("Instrument UI"=w503:refnum<class "Inst UI.MOTOR.lvclass">)
            n178 = call <vilib>:"Hide.vi"("error in (no error)"=w502, "SMO.UI"=w503) -> ("error out"=w501:errorcluster)  [unwired: 8 in, 1 out]
            n179 = call <vilib>:"Add State(s) to Queue__jki_lib_state_machine.vi"("State(s) in (\"\")"=w506) -> ("States Out"=w505:string)  [unwired: 14 in]
          }
          frame "Action: getAll" {
            n180 = Unbundle By Name(w510) -> ("getAll"=w507:T10, "Instrument"=w513:refnum<class "Inst.MOTOR.lvclass">)
            n181 = call "GET ALL.vim"("type"=w507, "error in (no error)"=w511, "Instrument in"=w513) -> ("error out"=w515:errorcluster, "getAll"=w508:T10, "Instrument out"=w509:refnum<class "Inst.MOTOR.lvclass">)  [unwired: 6 in]
            n182 = Bundle By Name(cluster=w510, "Instrument"=w509, "getAll"=w508) -> (w512:T12)
            n183 = call <vilib>:"Add State(s) to Queue__jki_lib_state_machine.vi"("State(s) in Front (\"\")"="" ("State(s) in Front (\"\")"), "State(s) in (\"\")"=w518) -> ("States Out"=w517:string)  [unwired: 13 in]
          }
          frame "Action: Open" {
            n184 = Unbundle By Name(w525) -> ("Instrument"=w523:refnum<class "Inst.MOTOR.lvclass">)
            n185 = call <userlib>:"Write Client Type.vi"("error in (no error)"=w520, "Client Type"=Client_Type--Enum."Local", "Instrument in"=w523) -> ("error out"=w521:errorcluster, "Instrument out"=w522:refnum<class "Inst.MOTOR.lvclass">)  [unwired: 7 in]
            n186 = call-dynamic "Open.vi"("error in (no error)"=w521, "Inst.MOTOR in"=w522) -> ("error out"=w528:errorcluster, "Inst.MOTOR out"=w524:refnum<class "Inst.MOTOR.lvclass">)  [unwired: 8 in]
            n187 = Bundle By Name(cluster=w525, "Instrument"=w524) -> (w526:T12)
            n188 = call <vilib>:"Add State(s) to Queue__jki_lib_state_machine.vi"("State(s) in Front (\"\")"="" ("State(s) in Front (\"\")"), "State(s) in (\"\")"=w531) -> ("States Out"=w530:string)  [unwired: 13 in]
          }
          frame "Action: Close" {
            n189 = Unbundle By Name(w533) -> ("Instrument"=w536:refnum<class "Inst.MOTOR.lvclass">)
            n190 = call-dynamic "Close.vi"("error in (no error)"=w534, "Inst.MOTOR in"=w536) -> ("error out"=w538:errorcluster, "Inst.MOTOR out"=w532:refnum<class "Inst.MOTOR.lvclass">)  [unwired: 8 in]
            n191 = Bundle By Name(cluster=w533, "Instrument"=w532) -> (w535:T12)
            n192 = call <vilib>:"Add State(s) to Queue__jki_lib_state_machine.vi"("State(s) in Front (\"\")"="" ("State(s) in Front (\"\")"), "State(s) in (\"\")"=w541) -> ("States Out"=w540:string)  [unwired: 13 in]
          }
          frame "Action: Send Message to Instrument" {
            # "Send a message (command, data, etc) to the Instrument:process.vi"
            n193 = Unbundle By Name(w548) -> ("Instrument"=w547:refnum<class "Inst.MOTOR.lvclass">, "Message.Command"=w543:string, "Message.Data"=w542:variant)
            n194 = call <userlib>:"Instrument.MessageToProcess.vi"("error in (no error)"=w545, "Data"=w542, "Command"=w543, "Instrument"=w547) -> ("error out"=w544:errorcluster, "Instrument out"=w546:refnum<class "Inst.MOTOR.lvclass">)  [unwired: 6 in]
            n195 = Bundle By Name(cluster=w548, "Instrument"=w546) -> (w549:T12)
            n196 = call <vilib>:"Add State(s) to Queue__jki_lib_state_machine.vi"("State(s) in Front (\"\")"="" ("State(s) in Front (\"\")"), "State(s) in (\"\")"=w553) -> ("States Out"=w552:string)  [unwired: 13 in]
          }
          frame "Action: Send Message to Child" {
            # "Send a message (command, data, etc) to the Instrument.Child:process.vi"
            n197 = Unbundle By Name(w558) -> ("Instrument"=w557:refnum<class "Inst.MOTOR.lvclass">)  [unwired: 1 out]
            n198 = call "Inst.MOTOR.MessageToProcess.vi"("error in (no error)"=w555, "Inst.MOTOR in"=w557) -> ("error out"=w554:errorcluster, "Inst.MOTOR out"=w556:refnum<class "Inst.MOTOR.lvclass">)  [unwired: 8 in]
            n199 = Bundle By Name(cluster=w558, "Instrument"=w556) -> (w559:T12)
            n200 = call <vilib>:"Add State(s) to Queue__jki_lib_state_machine.vi"("State(s) in Front (\"\")"="" ("State(s) in Front (\"\")"), "State(s) in (\"\")"=w563) -> ("States Out"=w562:string)  [unwired: 13 in]
          }
        }
      }
    }
    frame Error {
    }
  }
  n201 = call-parent "Process.vi"("error in"=w5, "Instrument UI in"=w4) -> ("error out"=w2:errorcluster, "Instrument UI out"=→"Inst UI.MOTOR out":refnum<class "Inst UI.MOTOR.lvclass">)  [unwired: 8 in]
  n202 = Merge Errors(w2, w1) -> (→"error out":errorcluster)
